vi "define.vi"(8 "error in (no error)":errorcluster, 11 "TrajectoryDL121017Hopping in":refnum<class "TrajectoryDL121017Hopping.lvclass">) -> (0 "error out":errorcluster, 3 "TrajectoryDL121017Hopping out":refnum<class "TrajectoryDL121017Hopping.lvclass">)   [LabVIEW 2010, in "TrajectoryDL121017Hopping.lvclass"]
doc: "Modal dialog on which the user can set the trajectory parameters."
uses:
  TrajectoryDL121017Hopping.lvclass
  common/xcontrols/XImage/XImage/XImage.xctl
  common/classes/ImageCollection/ImageCollection/ImageCollection.lvclass
  subpattern_type_enum.ctl
  common/xcontrols/XSettings/XSettings/XSettings.xctl
  common/classes/GenericComponent/GenericComponent/GenericComponent.lvclass
  TrajectoryDL121017Hopping.lvclass/TrajectoryDL121017Hopping.ctl
  <vilib>/Utility/miscctls.llb/LVPointTypeDef.ctl
  common/xcontrols/XImage/XImage/ROI_mode_enum.ctl
  common/classes/ImageCollection/ImageCollection/add_mode_enum.ctl
  common/classes/SpaceVector/SpaceVector/SpaceVector.lvclass
  common/classes/Image/Image/Image.lvclass
panel:
  out "effective no. of pixels":i32
  in  "hopping time":dbl[unit]=0.001 min=0.0 max=1.0
  in  "uncaging time":dbl[unit]=0.0005 min=0.0005 max=0.2
  out "repitition rate":dbl[unit]
  out "line scan time":dbl[unit]
  in  "total pixels":i32=10000 min=22 max=1000
  in  "button:enforceSettings":bool
  in  "XSettings":refnum<class "GenericComponent.lvclass">(xcontrol)
  in  "subpattern parameters tab":enum32{"spiral parameters"}(tab)
  in  "diameter":dbl[unit]=9.999999999999999e-06 min=0.0 max=0.0005
  in  "number of windings":i32=1 min=1
  in  "button:recreateTrajectory":bool
  in  "subpattern type":T1
  in  "button:cancel":bool
  in  "button:ok":bool
  in  "XImage":refnum<class "ImageCollection.lvclass">(xcontrol)
  # "Define Trajectory"
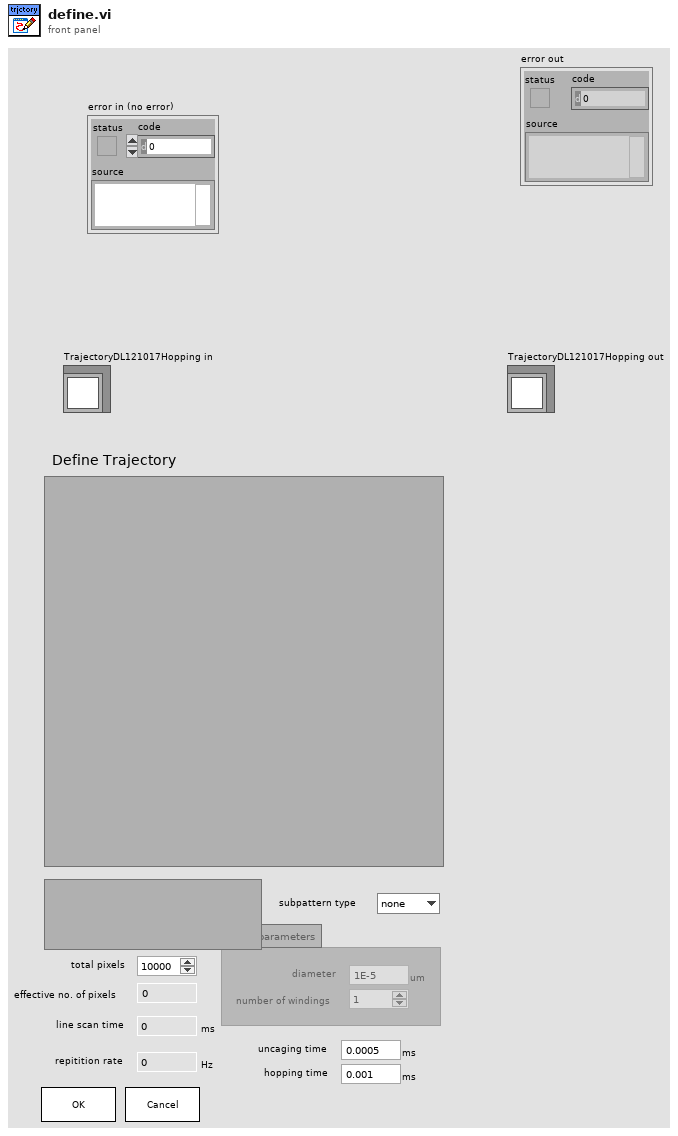
[diagram p1: front panel]
types:
  T1 = typedef "TrajectoryDL121017Hopping.lvclass/subpattern_type_enum.ctl" = enum16{"none", "spiral"}
  T2 = typedef "LVPointTypeDef.ctl" = cluster{"Horizontal":i16, "Vertical":i16}
  T3 = cluster{"Zoom Tool":bool, "Selection Tool":bool, "Pan Tool":bool, "Point Tool":bool, "Line Tool":bool, "Rectangle Tool":bool, "Rotated Rectangle Tool":bool, "Polyline Tool":bool, "Polygon Tool":bool, "Freehand Tool":bool, "Closed Freehand Tool":bool, "Ellipse Tool":bool, "Annulus Tool":bool}
  T4 = typedef "XImage.xctl/ROI_mode_enum.ctl" = enum16{"none", "IMAQROIs", "PointCollection"}
  T5 = typedef "ImageCollection.lvclass/add_mode_enum.ctl" = enum16{"instance", "copy"}
  T6 = enum8{"Enabled", "Disabled", "Disabled and Grayed Out"}
  T7 = typedef "XImage.xctl/ROImicrons_frames_cluster.ctl" = cluster{"ROI":T8[]}
  T8 = typedef "ROImicrons_cluster.ctl" = cluster{"Global Rectangle":dbl[unit][], "Contours":cluster{"Contour Type":u32, "ROI Type":u32, "Points":dbl[unit][]}[]}
  T9 = typedef "XImage.xctl/last_action_enum.ctl" = enum16{"not specified", "image loaded", "frame changed", "ROIs changed"}
  T10 = cluster{"Contour Type":u32, "ROI Type":u32, "Points":dbl[unit][]}[]
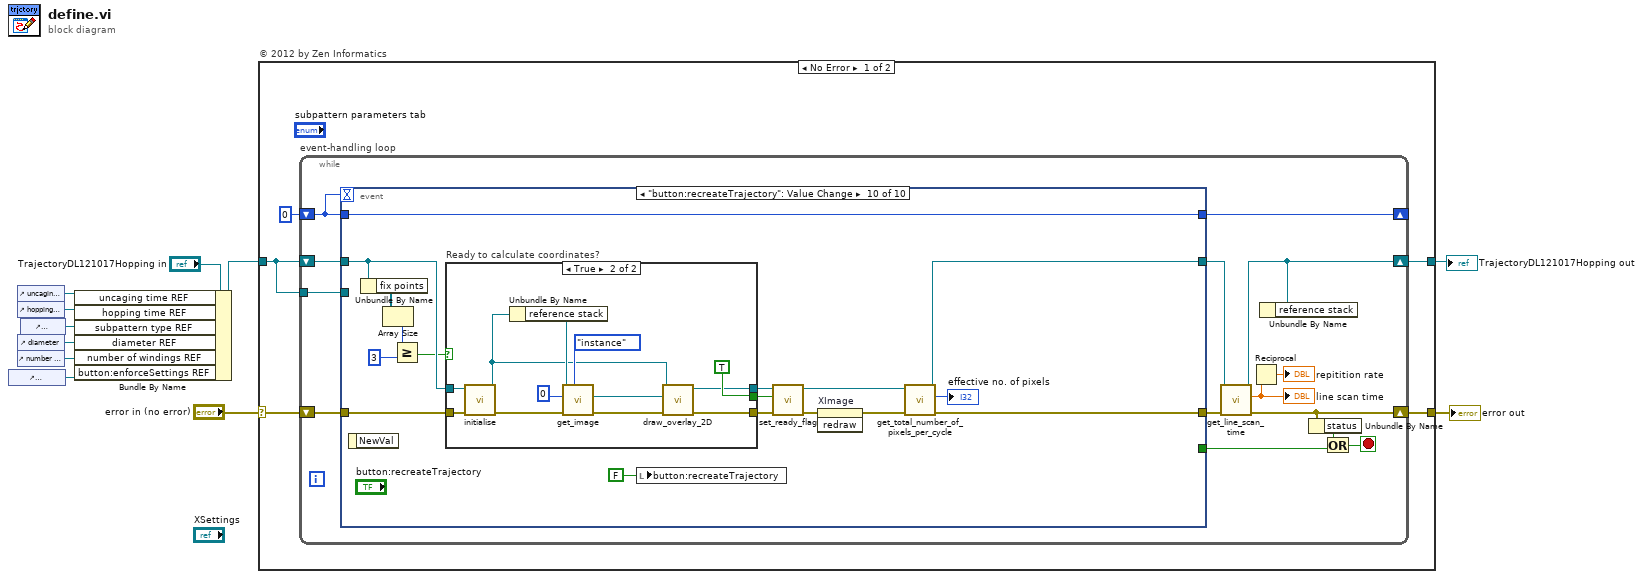
[diagram p0: block diagram]
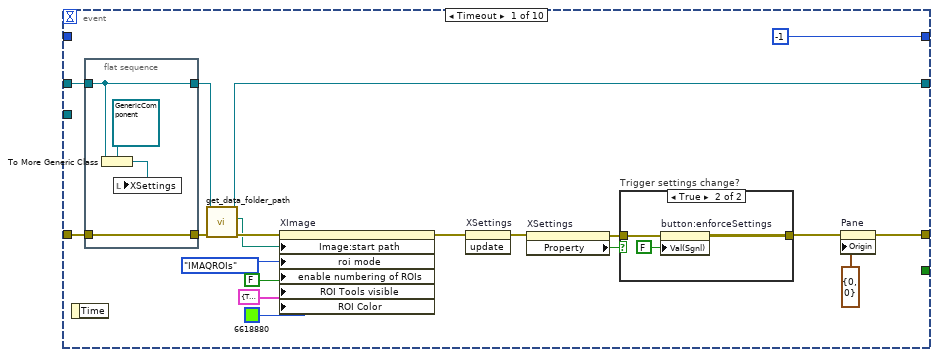
[diagram p2: hidden frame]
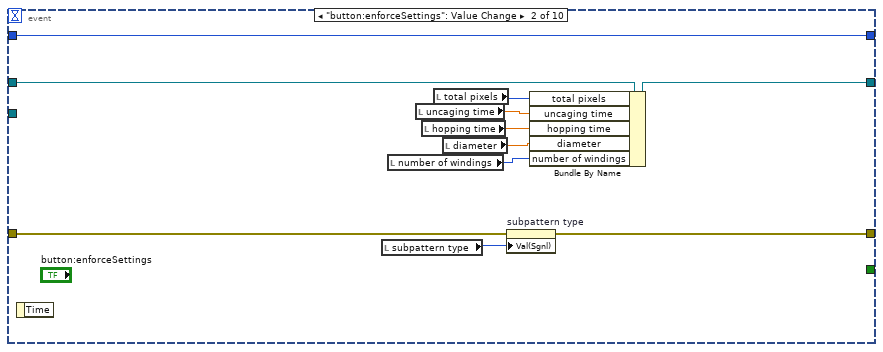
[diagram p4: hidden frame]
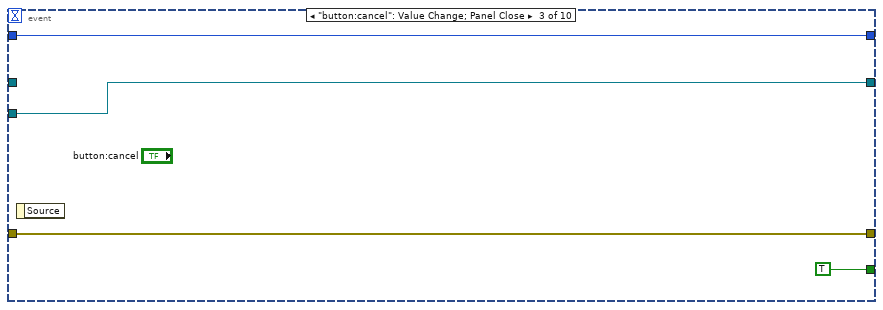
[diagram p5: hidden frame]
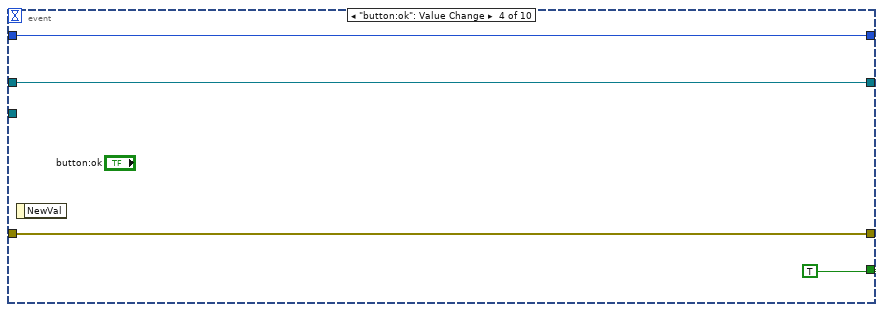
[diagram p6: hidden frame]
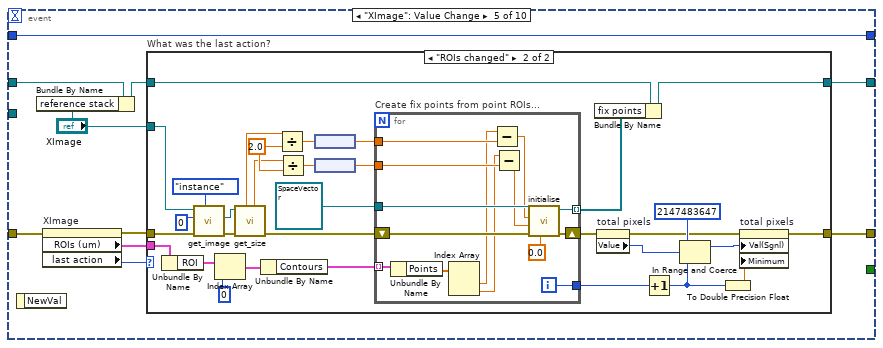
[diagram p7: hidden frame]
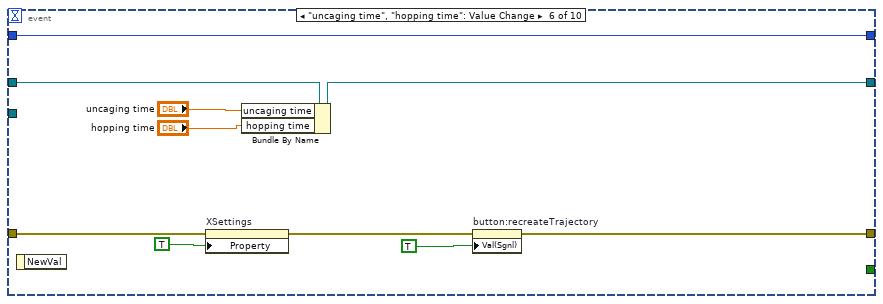
[diagram p9: hidden frame]
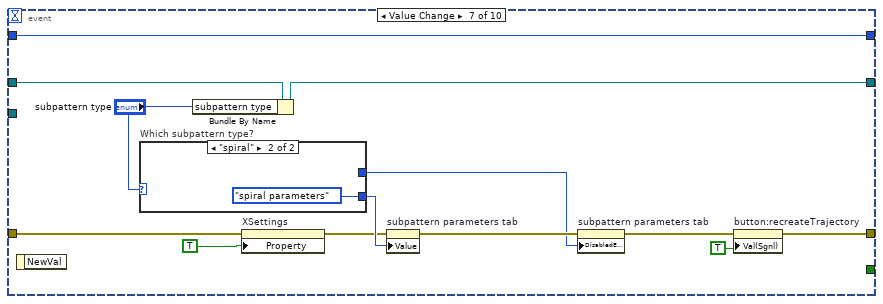
[diagram p10: hidden frame]
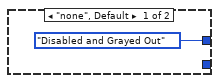
[diagram p11: hidden frame]
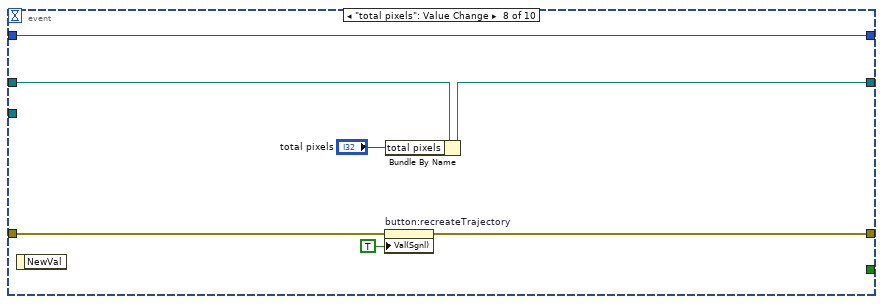
[diagram p12: hidden frame]
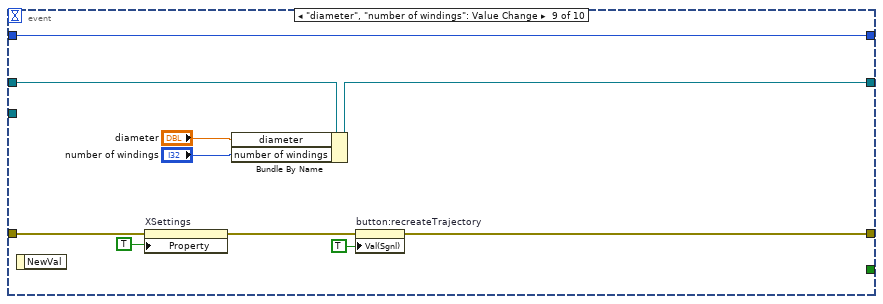
[diagram p13: hidden frame]
diagram:
  n1 = control-ref of="button:enforceSettings"() -> (w1:refnum<vi>)
  n2 = control-ref of="uncaging time"() -> (w2:refnum<vi>)
  n3 = control-ref of="hopping time"() -> (w3:refnum<vi>)
  n4 = control-ref of="diameter"() -> (w5:refnum<vi>)
  n5 = control-ref of="number of windings"() -> (w6:refnum<vi>)
  n6 = control-ref of="subpattern type"() -> (w4:refnum<vi>)
  n7 = Bundle By Name(cluster="TrajectoryDL121017Hopping in", "uncaging time REF"=w2, "hopping time REF"=w3, "subpattern type REF"=w4, "diameter REF"=w5, "number of windings REF"=w6, "button:enforceSettings REF"=w1) -> (w7:refnum<class "TrajectoryDL121017Hopping.lvclass">)
  n8 = case "© 2012 by Zen Informatics" shown="No Error" "error in (no error)" {
    selector: "error in (no error)" -> [w16 w208]
    tunnel: w7 -> [w12 w209]
    tunnel: [w15 w208] -> w10
    tunnel: [w14 w209] -> w9
    frame No Error {
      n9 = while "event-handling loop" {
        shift-right: [w22] -> w15
        shift-left: w16 -> [w29]
        shift-right: [w17] -> w14
        shift-left: w12 -> [w30]
        shift-right: [w24] -> _
        shift-left: 0 -> [w25]
        tunnel: w12 -> [w23]
        stop <- w26 stop-if-true
        n10 = event shown="[9] \"button:recreateTrajectory\": Value Change" {
          selector: _ -> [_ _ _ _ _ _ _ _ _ _]
          dyn-events: _ -> [_ _ _ _ _ _ _ _ _ _]
          timeout: w25 -> [_ _ _ _ _ _ _ _ _ _]
          tunnel: w30 -> [w44 w67 _ w76 w79 w143 w156 w165 w173 w188]
          tunnel: w29 -> [w43 w60 w72 w75 w85 w136 w146 w161 w168 w192]
          tunnel: [w33 w58 w72 w75 w77 w138 w151 w160 w170 w180] -> w21
          tunnel: [w35 w66 w69 w76 w78 w142 w155 w164 w172 w178] -> w20
          tunnel: [_ _ TRUE TRUE _ _ _ _ _ _] -> w28
          tunnel: [-1 w68 w70 w73 w86 w144 w157 w166 w176 w193] -> w24
          tunnel: w25 -> [_ w68 w70 w73 w86 w144 w157 w166 w176 w193]
          tunnel: w23 -> [_ _ w69 _ _ _ _ _ _ _]
          event Timeout {
            n11 = event-data() -> ()  [unwired: 1 in, 1 out]
            n12 = flat-sequence {
              tunnel: w44 -> [w54]
              tunnel: [w55] -> w42
              tunnel: w43 -> [w55]
              tunnel: [w54] -> w41
              frame #0 {
                n13 = To More Generic Class(target class=refnum<class "GenericComponent.lvclass"> refnum ("GenericComponent.lvclass"), reference=w54) -> (generic class reference=w56:refnum<class "GenericComponent.lvclass">)
                n14 = local write "XSettings"(w56) -> ()
              }
            }
            n15 = call-dynamic "get_data_folder_path.vi"("error in (no error)"=w42, "GenericComponent in"=w41) -> ("error out"=w45:errorcluster, "data folder path"=w39:path, "GenericComponent out"=w35:refnum<class "TrajectoryDL121017Hopping.lvclass">)  [unwired: 7 in]
            n16 = property on="XImage" class="XImage (strict)"(error in=w45, "Image:start path"=w39, "roi mode"=ROI_mode_enum."IMAQROIs" ("ROI:mode"), "enable numbering of ROIs"=FALSE ("ROI:enable numbering of ROIs"), "ROI Tools visible"=T3 {"Zoom Tool"=TRUE, "Selection Tool"=TRUE, "Pan Tool"=TRUE, "Point Tool"=TRUE, "Line Tool"=FALSE, "Rectangle Tool"=FALSE, "Rotated Rectangle Tool"=FALSE, "Polyline Tool"=FALSE, "Polygon Tool"=FALSE, "Freehand Tool"=FALSE, "Closed Freehand Tool"=FALSE, "Ellipse Tool"=FALSE, "Annulus Tool"=FALSE} ("ROI:ROI Tools Palette visible"), "ROI Color"=u32 6618880) -> (error out=w34:errorcluster)  [unwired: 1 in, 1 out]
            n17 = invoke on="XSettings" class="XSettings (strict)" method="update"(error in=w34) -> (error out=w38:errorcluster)  [unwired: 2 in, 2 out]
            n18 = property on="XSettings" class="XSettings (strict)"(error in=w38) -> (error out=w37:errorcluster, "Property"=w36:bool)  [unwired: 1 in, 1 out]
            n19 = case "Trigger settings change?" shown="True" w36 {
              tunnel: w37 -> [w50 w53]
              tunnel: [w50 w51] -> w32
              frame False {
              }
              frame True {
                n20 = property on="button:enforceSettings" class="Bool (strict)"(error in=w53, "Val(Sgnl)"=FALSE ("Value (Signaling)")) -> (error out=w51:errorcluster)  [unwired: 1 in, 1 out]
              }
            }
            n21 = property on="Pane" class="Pane"(error in=w32, "Origin"=T2 {"Horizontal"=0, "Vertical"=0}) -> (error out=w33:errorcluster)  [unwired: 1 in, 1 out]
          }
          event "button:enforceSettings": Value Change {
            n22 = event-data() -> ()  [unwired: 1 in, 1 out]
            n23 = local read "subpattern type"() -> (w59:T1)
            n24 = local read "number of windings"() -> (w62:i32)
            n25 = local read "uncaging time"() -> (w65:dbl[unit])
            n26 = local read "hopping time"() -> (w64:dbl[unit])
            n27 = local read "total pixels"() -> (w61:i32)
            n28 = local read "diameter"() -> (w63:dbl[unit])
            n29 = property on="subpattern type" class="Enum (strict)"(error in=w60, "Val(Sgnl)"=w59) -> (error out=w58:errorcluster)  [unwired: 1 in, 1 out]
            n30 = Bundle By Name(cluster=w67, "total pixels"=w61, "uncaging time"=w65, "hopping time"=w64, "diameter"=w63, "number of windings"=w62) -> (w66:refnum<class "TrajectoryDL121017Hopping.lvclass">)
          }
          event "button:cancel": Value Change; Panel Close {
            n31 = event-data() -> ()  [unwired: 1 in, 1 out]
          }
          event "button:ok": Value Change {
            n32 = event-data() -> ()  [unwired: 1 in, 1 out]
          }
          event "XImage": Value Change {
            n33 = event-data() -> ()  [unwired: 1 in, 1 out]
            n34 = Bundle By Name(cluster=w79, "reference stack"="XImage") -> (w83:refnum<class "TrajectoryDL121017Hopping.lvclass">)
            n35 = property on="XImage" class="XImage (strict)"(error in=w85) -> (error out=w80:errorcluster, "ROIs (um)"=w81:T7, "last action"=w84:T9)  [unwired: 1 in, 1 out]
            n36 = case "What was the last action?" shown="\"ROIs changed\"" w84 {
              tunnel: w80 -> [w88 w103]
              tunnel: [w88 w96] -> w77
              tunnel: w83 -> [w87 w102]
              tunnel: [w87 w98] -> w78
              tunnel: "XImage" -> [_ w101]
              tunnel: w81 -> [_ w99]
              frame Default {
              }
              frame "ROIs changed" {
                w116 = 2.0 ("y")
                n37 = Unbundle By Name(w99) -> ("ROI"=w104:T8[])
                n38 = call-dynamic "get_image.vi"("get image as..."=add_mode_enum."instance", "error in (no error)"=w103, "index"=0, "ImageCollection in"=w101) -> ("error out"=w111:errorcluster, "Image.lvclass"=w113:refnum<class "Image.lvclass">)  [unwired: 5 in, 1 out]
                n39 = Index Array(array=w104, index=0) -> (element=w106:T8)
                n40 = call-dynamic "get_size.vi"("error in (no error)"=w111, "Image in"=w113) -> ("error out"=w112:errorcluster, "physical size y"=w115:dbl, "physical size x"=w114:dbl)  [unwired: 2 in, 5 out]
                n41 = Unbundle By Name(w106) -> ("Contours"=w107:T10)
                n42 = Divide(x=w114, y=w116) -> (x/y=w117:dbl)
                n43 = Divide(x=w115, y=w116) -> (x/y=w118:dbl)
                n44 = node(w117) -> (w119:dbl[unit])
                n45 = node(w118) -> (w120:dbl[unit])
                n46 = for "Create fix points from point ROIs..." {
                  tunnel: w107 -> [w130] mode=indexing
                  shift-right: [w132] -> w91
                  shift-left: w112 -> [w134]
                  tunnel: refnum<class "SpaceVector.lvclass"> refnum ("SpaceVector.lvclass") -> [w133]
                  tunnel: [w131] -> w109 mode=indexing
                  tunnel: w119 -> [w127]
                  tunnel: w120 -> [w126]
                  tunnel: [w121] -> w97
                  i -> [w121]
                  n47 = Unbundle By Name(w130) -> ("Points"=w128:dbl[unit][])
                  n48 = Index Array(array=w128) -> (element #1=w123:dbl[unit], element #2=w125:dbl[unit])  [unwired: 2 in]
                  n49 = Subtract(x=w123, y=w127) -> (x-y=w122:dbl[unit])
                  n50 = Subtract(x=w125, y=w126) -> (x-y=w124:dbl[unit])
                  n51 = call "initialise.vi"("z"=dbl[unit] 0.0, "error in (no error)"=w134, "y"=w124, "x"=w122, "SpaceVector in"=w133) -> ("error out"=w132:errorcluster, "SpaceVector out"=w131:refnum<class "SpaceVector.lvclass">)  [unwired: 5 in]
                }
                n52 = Bundle By Name(cluster=w102, "fix points"=w109) -> (w98:refnum<class "TrajectoryDL121017Hopping.lvclass">)
                n53 = property on="total pixels" class="DigNum (strict)"(error in=w91) -> (error out=w90:errorcluster, "Value"=w89:i32)  [unwired: 1 in, 1 out]
                n54 = Increment(x=w97) -> (x+1=w92:i32)
                n55 = In Range and Coerce(upper limit=2147483647, x=w89, lower limit=w92) -> (coerced(x)=w93:i32)  [unwired: 1 out]
                n56 = To Double Precision Float(number=w92) -> (double precision float=w94:dbl)
                n57 = property on="total pixels" class="DigNum (strict)"(error in=w90, "Val(Sgnl)"=w93, "Minimum"=w94) -> (error out=w96:errorcluster)  [unwired: 1 in, 1 out]
              }
            }
          }
          event "uncaging time", "hopping time": Value Change {
            n58 = event-data() -> ()  [unwired: 1 in, 1 out]
            n59 = property on="XSettings" class="XSettings (strict)"(error in=w136, "Property"=TRUE ("is user-defined?")) -> (error out=w135:errorcluster)  [unwired: 1 in, 1 out]
            n60 = Bundle By Name(cluster=w143, "uncaging time"="uncaging time", "hopping time"="hopping time") -> (w142:refnum<class "TrajectoryDL121017Hopping.lvclass">)
            n61 = property on="button:recreateTrajectory" class="Bool (strict)"(error in=w135, "Val(Sgnl)"=TRUE ("Value (Signaling)")) -> (error out=w138:errorcluster)  [unwired: 1 in, 1 out]
          }
          event Value Change {
            n62 = event-data() -> ()  [unwired: 1 in, 1 out]
            n63 = case "Which subpattern type?" shown="\"spiral\"" "subpattern type" {
              tunnel: [_ enum32{"spiral parameters"}."spiral parameters" ("subpattern parameters tab")] -> w153
              tunnel: [T6."Disabled and Grayed Out" ("Disabled") _] -> w148
              frame "none", Default {
              }
              frame "spiral" {
              }
            }
            n64 = Bundle By Name(cluster=w156, "subpattern type"="subpattern type") -> (w155:refnum<class "TrajectoryDL121017Hopping.lvclass">)
            n65 = property on="XSettings" class="XSettings (strict)"(error in=w146, "Property"=TRUE ("is user-defined?")) -> (error out=w145:errorcluster)  [unwired: 1 in, 1 out]
            n66 = property on="subpattern parameters tab" class="TabCtl (strict)"(error in=w145, "Value"=w153) -> (error out=w150:errorcluster)  [unwired: 1 in, 1 out]
            n67 = property on="subpattern parameters tab" class="TabCtl (strict)"(error in=w150, "DisabledEnum"=w148) -> (error out=w149:errorcluster)  [unwired: 1 in, 1 out]
            n68 = property on="button:recreateTrajectory" class="Bool (strict)"(error in=w149, "Val(Sgnl)"=TRUE ("Value (Signaling)")) -> (error out=w151:errorcluster)  [unwired: 1 in, 1 out]
          }
          event "total pixels": Value Change {
            n69 = event-data() -> ()  [unwired: 1 in, 1 out]
            n70 = property on="button:recreateTrajectory" class="Bool (strict)"(error in=w161, "Val(Sgnl)"=TRUE ("Value (Signaling)")) -> (error out=w160:errorcluster)  [unwired: 1 in, 1 out]
            n71 = Bundle By Name(cluster=w165, "total pixels"="total pixels") -> (w164:refnum<class "TrajectoryDL121017Hopping.lvclass">)
          }
          event "diameter", "number of windings": Value Change {
            n72 = event-data() -> ()  [unwired: 1 in, 1 out]
            n73 = property on="XSettings" class="XSettings (strict)"(error in=w168, "Property"=TRUE ("is user-defined?")) -> (error out=w167:errorcluster)  [unwired: 1 in, 1 out]
            n74 = Bundle By Name(cluster=w173, "diameter"="diameter", "number of windings"="number of windings") -> (w172:refnum<class "TrajectoryDL121017Hopping.lvclass">)
            n75 = property on="button:recreateTrajectory" class="Bool (strict)"(error in=w167, "Val(Sgnl)"=TRUE ("Value (Signaling)")) -> (error out=w170:errorcluster)  [unwired: 1 in, 1 out]
          }
          event "button:recreateTrajectory": Value Change {
            n76 = event-data() -> ()  [unwired: 1 in, 1 out]
            n77 = Unbundle By Name(w188) -> ("fix points"=w187:refnum<class "SpaceVector.lvclass">[])
            n78 = Array Size(array=w187) -> (size(s)=w186:i32)
            n79 = Greater Or Equal?(x=w186, y=3) -> (x >= y?=w184:bool)
            n80 = case "Ready to calculate coordinates?" shown="True" w184 {
              tunnel: w192 -> [w194 w204]
              tunnel: [w195 w197] -> w190
              tunnel: w188 -> [w195 w200]
              tunnel: [w194 w196] -> w191
              tunnel: [_ TRUE] -> w189
              frame False {
              }
              frame True {
                n81 = call-dynamic "initialise.vi"("error in (no error)"=w204, "GenericTrajectory in"=w200) -> ("error out"=w203:errorcluster, "GenericTrajectory out"=w201:refnum<class "TrajectoryDL121017Hopping.lvclass">)  [unwired: 8 in]
                n82 = Unbundle By Name(w201) -> ("reference stack"=w206:refnum<class "ImageCollection.lvclass">)
                n83 = call-dynamic "get_image.vi"("get image as..."=add_mode_enum."instance", "error in (no error)"=w203, "index"=0, "ImageCollection in"=w206) -> ("error out"=w202:errorcluster, "Image.lvclass"=w199:refnum<class "Image.lvclass">)  [unwired: 5 in, 1 out]
                n84 = call-dynamic "draw_overlay_2D.vi"("error in (no error)"=w202, "image in"=w199, "GenericTrajectory in"=w201) -> ("error out"=w196:errorcluster, "GenericTrajectory out"=w197:refnum<class "TrajectoryDL121017Hopping.lvclass">)  [unwired: 6 in, 1 out]
              }
            }
            n85 = local write "button:recreateTrajectory"(FALSE ("button:recreateTrajectory")) -> ()
            n86 = call-dynamic "set_ready_flag.vi"("error in (no error)"=w191, "ready for initialisation?"=w189, "GenericTrajectory in"=w190) -> ("error out"=w183:errorcluster, "GenericTrajectory out"=w179:refnum<class "TrajectoryDL121017Hopping.lvclass">)  [unwired: 7 in]
            n87 = invoke on="XImage" class="XImage (strict)" method="redraw"(error in=w183) -> (error out=w181:errorcluster)  [unwired: 2 in, 2 out]
            n88 = call-dynamic "get_total_number_of_pixels_per_cycle.vi"("error in (no error)"=w181, "GenericTrajectory in"=w179) -> ("error out"=w180:errorcluster, "total number of pixels per cycle"=→"effective no. of pixels":i32, "GenericTrajectory out"=w178:refnum<class "TrajectoryDL121017Hopping.lvclass">)  [unwired: 7 in]
          }
        }
        n89 = call "get_line_scan_time.vi"("error in (no error)"=w21, "TrajectoryDL121017Hopping in"=w20) -> ("error out"=w22:errorcluster, "line scan time"=w19:dbl[unit], "TrajectoryDL121017Hopping out"=w17:refnum<class "TrajectoryDL121017Hopping.lvclass">)  [unwired: 7 in]
        "line scan time" <- w19
        n90 = Reciprocal(x=w19) -> (1/x=→"repitition rate":dbl[unit])
        n91 = Unbundle By Name(w17) -> ()  [unwired: 1 out]
        n92 = Unbundle By Name(w22) -> ("status"=w27:bool)
        n93 = Or(x=w27, y=w28) -> (x .or. y?=w26:bool)
      }
    }
    frame Error {
    }
  }
  "error out" <- w10
  "TrajectoryDL121017Hopping out" <- w9
